vi "Dense Layer.vi"(9 "Bias (1xb)":dbl[](array[numeric]), 10 "Data X (1xa)":dbl[](array[numeric]), 11 "Weights (axb)":dbl[][](array[numeric])) -> (2 "Output Y (1xb)":dbl[](array[numeric]))   [LabVIEW 2018]
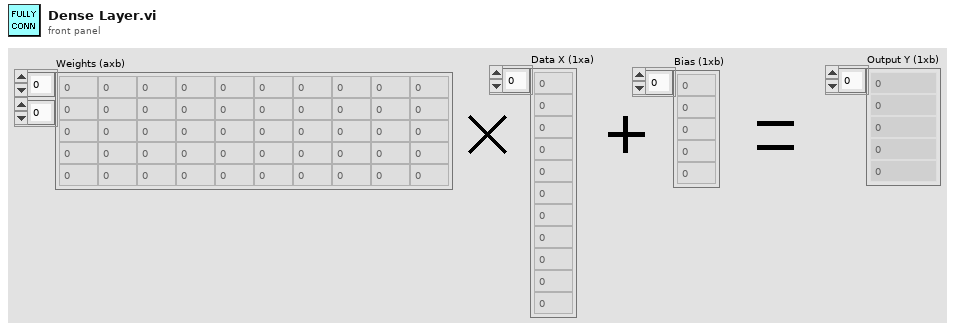
[diagram p1: front panel]
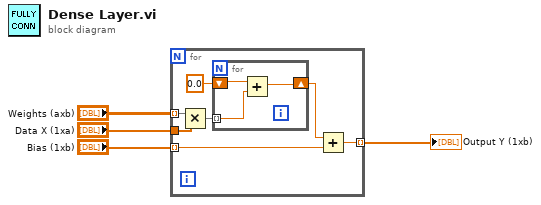
[diagram p0: block diagram]
diagram:
  n1 = for {
    tunnel: "Weights (axb)" -> [w8] mode=indexing
    tunnel: "Data X (1xa)" -> [w9]
    tunnel: "Bias (1xb)" -> [w11] mode=indexing
    tunnel: [w10] -> w1 mode=indexing
    n2 = Multiply(x=w8, y=w9) -> (x*y=w7:dbl[])
    n3 = for {
      tunnel: w7 -> [w14] mode=indexing
      shift-right: [w12] -> w5
      shift-left: sgl 0.0 -> [w13]
      n4 = Add(x=w13, y=w14) -> (x+y=w12:dbl)
    }
    n5 = Add ("Add.vi")(x=w5, y=w11) -> (x+y=w10:dbl)
  }
  "Output Y (1xb)" <- w1
